vi "Reset.vi"(8 "error in (no error)":errorcluster, 11 "Debug State Analyzer in":refnum<class "Debug State Analyzer.lvclass">) -> (0 "error out":errorcluster, 3 "Debug State Analyzer out":refnum<class "Debug State Analyzer.lvclass">)   [LabVIEW 2020, in "Debug State Analyzer.lvclass"]
uses:
  Debug State Analyzer.lvclass
  Debug State Analyzer.lvclass/Debug State Analyzer.ctl
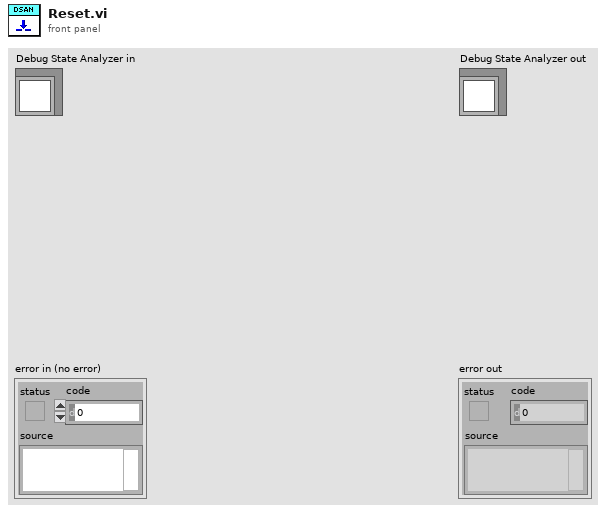
[diagram p1: front panel]
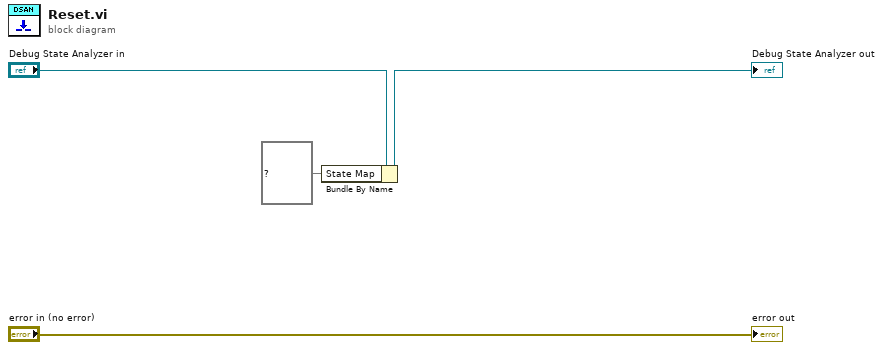
[diagram p0: block diagram]
diagram:
  n1 = Bundle By Name(cluster="Debug State Analyzer in", "State Map"=map{string, string} {}) -> (→"Debug State Analyzer out":refnum<class "Debug State Analyzer.lvclass">)
  "error out" <- "error in (no error)"
